vi "ex 2.vi"() -> ()   [LabVIEW 2019]
panel:
  out "rouge2":bool
  out "jaune 2":bool
  out "vert 2":bool
  in  "si imbriqué":dbl(slide) scale=0.0..12.0
  out "rouge":bool
  out "jaune":bool
  out "vert":bool
  in  "si  simple":dbl(slide) scale=0.0..12.0
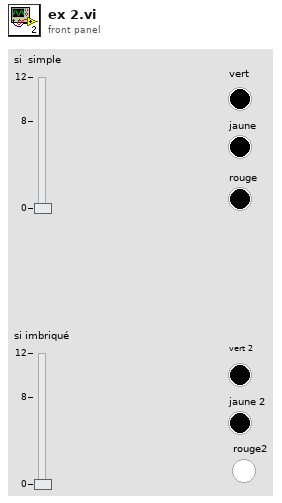
[diagram p1: front panel]
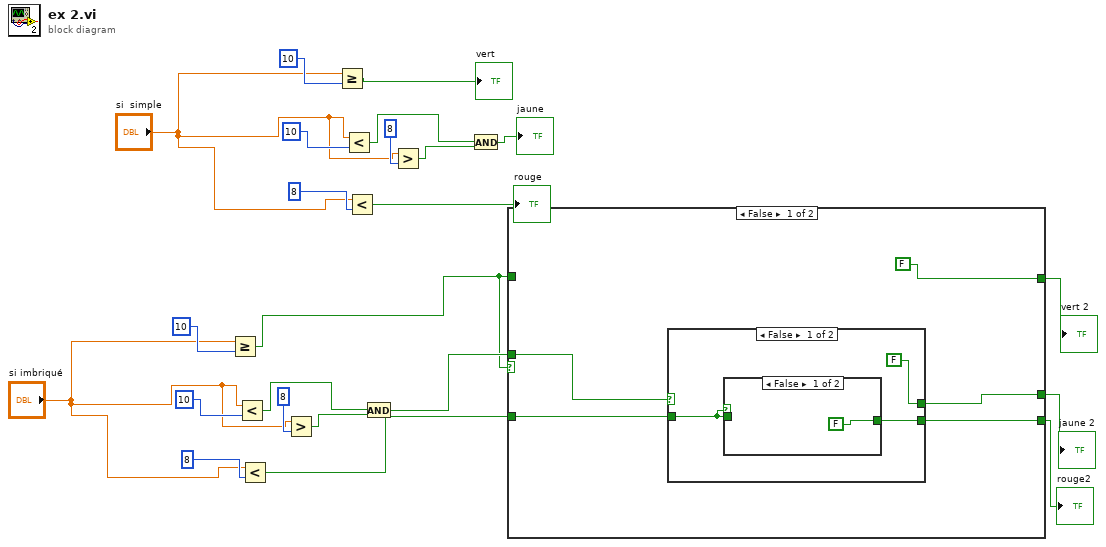
[diagram p0: block diagram]
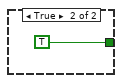
[diagram p2: hidden frame]
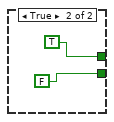
[diagram p3: hidden frame]
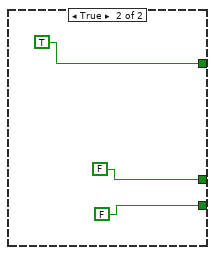
[diagram p4: hidden frame]
diagram:
  n1 = Greater Or Equal?(x="si imbriqué", y=10) -> (x >= y?=w1:bool)
  n2 = Less?(x="si imbriqué", y=10) -> (x < y?=w12:bool)
  n3 = Less?(x="si imbriqué", y=8) -> (x < y?=w3:bool)
  n4 = Greater?(x="si imbriqué", y=8) -> (0:w13:bool)
  n5 = Greater Or Equal?(x="si  simple", y=10) -> (x >= y?=→"vert":bool)
  n6 = Less?(x="si  simple", y=10) -> (x < y?=w20:bool)
  n7 = Less?(x="si  simple", y=8) -> (x < y?=→"rouge":bool)
  n8 = And(x=w12, y=w13) -> (x .and. y?=w5:bool)
  n9 = Greater?(x="si  simple", y=8) -> (0:w21:bool)
  n10 = And(x=w20, y=w21) -> (x .and. y?=→"jaune":bool)
  n11 = case shown="False" w1 {
    tunnel: [FALSE TRUE] -> w6
    tunnel: w1 -> [_ _]
    tunnel: w5 -> [w28 _]
    tunnel: [w27 FALSE] -> w4
    tunnel: w3 -> [w25 _]
    tunnel: [w24 FALSE] -> w2
    frame False {
      n12 = case shown="False" w28 {
        tunnel: [FALSE TRUE] -> w27
        tunnel: w25 -> [w29 _]
        tunnel: [w30 FALSE] -> w24
        frame False {
          n13 = case shown="False" w29 {
            tunnel: w29 -> [_ _]
            tunnel: [FALSE TRUE] -> w30
            frame False {
            }
            frame True {
            }
          }
        }
        frame True {
        }
      }
    }
    frame True {
    }
  }
  "vert 2" <- w6
  "jaune 2" <- w4
  "rouge2" <- w2
